vi "Error.Remove Duplicate Errors.vi"(11 "Errors In":errorcluster[](array[cluster])) -> (3 "Errors Out":errorcluster[](array[cluster]))   [LabVIEW 2018]
panel:
  # "Remove Dup Error"
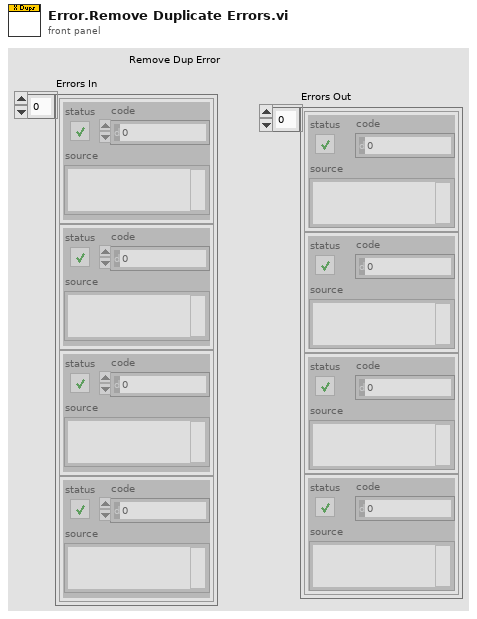
[diagram p1: front panel]
types:
  T1 = cluster{"status":bool, "code":bool, "source":bool}
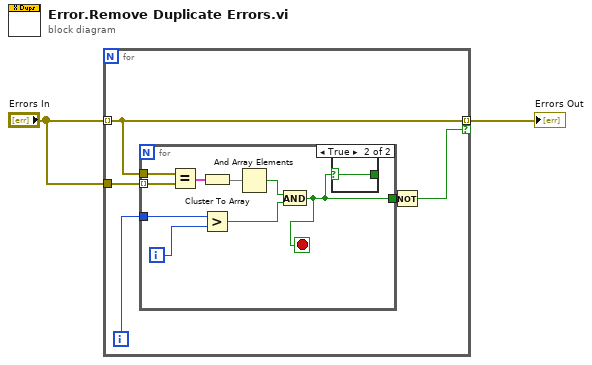
[diagram p0: block diagram]
diagram:
  n1 = for {
    tunnel: "Errors In" -> [w6] mode=indexing
    tunnel: [w6] -> w1 mode=indexing if=w3
    tunnel: "Errors In" -> [w7]
    i -> [w5]
    n2 = for {
      tunnel: w7 -> [w16] mode=indexing
      tunnel: w6 -> [w15]
      tunnel: w5 -> [w9]
      tunnel: [w8] -> w4
      i -> [w10]
      stop <- w8 stop-if-true
      n3 = Equal?(x=w15, y=w16) -> (x = y?=w14:T1)
      n4 = Cluster To Array(cluster=w14) -> (array=w12:bool[])
      n5 = Greater?(x=w9, y=w10) -> (0:w11:bool)
      n6 = And Array Elements(Boolean array=w12) -> (logical AND=w13:bool)
      n7 = And(x=w13, y=w11) -> (x .and. y?=w8:bool)
      n8 = case shown="True" w8 {
        selector: w8 -> [_ w17]
        tunnel: [_ w17] -> _
        frame False {
        }
        frame True {
        }
      }
    }
    n9 = Not(x=w4) -> (.not. x?=w3:bool)
  }
  "Errors Out" <- w1
